vi "rad_Check IF LinuxRT.vi"(8 "Error In":errorcluster, 11 "System Session In":refnum<k21>="RAD-Test-9068 (169.254.113.8)") -> (0 "Error Out":errorcluster, 2 "Target is LinuxRT?":bool, 3 "System Session Out":refnum<k21>="RAD-Test-9068 (169.254.113.8)", 4 "Target is ARMv7?":bool, 6 "Target is Intel x64?":bool)   [LabVIEW 2023]
uses:
  <resource>/objmgr/nisysapi.rc
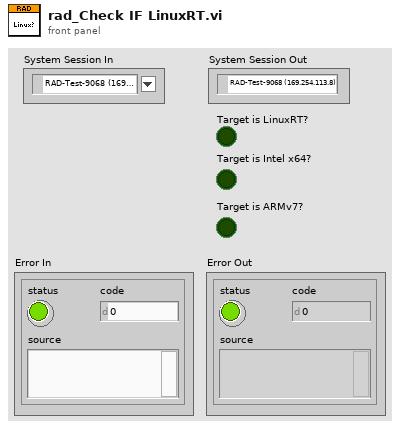
[diagram p1: front panel]
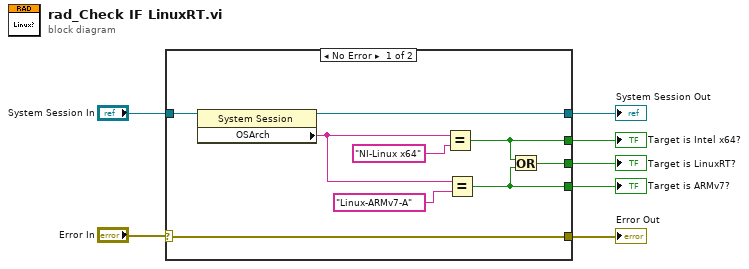
[diagram p0: block diagram]
diagram:
  n1 = case shown="No Error" "Error In" {
    selector: "Error In" -> [w14 w18]
    tunnel: "System Session In" -> [w16 w17]
    tunnel: [w15 w17] -> w6
    tunnel: [w10 _] -> w5
    tunnel: [w8 _] -> w4
    tunnel: [w14 w18] -> w2
    tunnel: [w9 _] -> w1
    frame No Error {
      n2 = property class="System Session"(reference=w16) -> (reference out=w15:refnum<k21>, "OSArch"=w13:string)  [unwired: 1 in, 1 out]
      n3 = Equal?(x=w13, y="NI-Linux x64") -> (x = y?=w9:bool)
      n4 = Equal?(x=w13, y="Linux-ARMv7-A") -> (x = y?=w8:bool)
      n5 = Or(x=w9, y=w8) -> (x .or. y?=w10:bool)
    }
    frame Error {
    }
  }
  "Target is LinuxRT?" <- w5
  "Target is Intel x64?" <- w1
  "Target is ARMv7?" <- w4
  "System Session Out" <- w6
  "Error Out" <- w2
